vi "Set Output Mode.vi"(8 "error in (no error)":errorcluster caption="错误输入（无错误）", 10 "Output Mode":u32(ring) items=["Standby", "Operate"], 11 "多功能校准源接口 输入":refnum<class "多功能校准源接口.lvclass">) -> (0 "error out":errorcluster caption="错误输出", 3 "多功能校准源接口 输出":refnum<class "多功能校准源接口.lvclass">)   [LabVIEW 2020, in "多功能校准源接口.lvlib" / "多功能校准源接口.lvclass"]
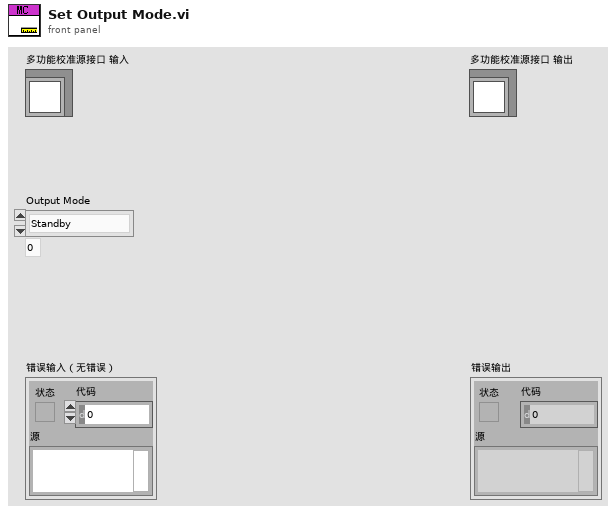
[diagram p1: front panel]
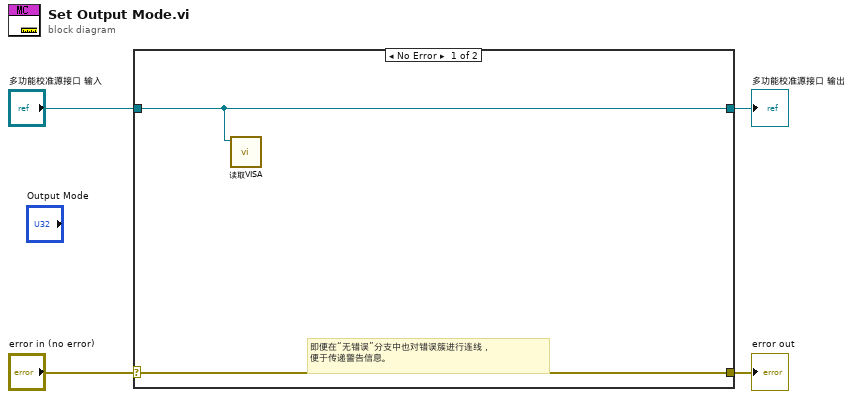
[diagram p0: block diagram]
diagram:
  n1 = case shown="No Error" "error in (no error)" {
    selector: "error in (no error)" -> [w6 w8]
    tunnel: [w6 w8] -> w3
    tunnel: [w5 w7] -> w1
    tunnel: "多功能校准源接口 输入" -> [w5 w7]
    frame No Error {
      # "即便在“无错误”分支中也对错误簇进行连线，\n便于传递警告信息。"
      n2 = call "读取VISA.vi"("多功能校准源接口输入"=w5) -> ()  [unwired: 8 in, 3 out]
    }
    frame Error {
    }
  }
  "error out" <- w3
  "多功能校准源接口 输出" <- w1
